vi "1D ARRAY TO 2D ARRAY.vi"() -> ()   [LabVIEW 2017]
panel:
  out "deleted portion":dbl[](array[numeric])
  out "array w/ subset deleted":dbl[](array[numeric])
  out "output array":dbl[](array[numeric])
  in  "new element/subarray":dbl
  out "subarray":dbl[](array[numeric])
  out "appended array":dbl[][](array[numeric])
  in  "Array 2":dbl[](array[numeric])
  in  "Array":dbl[](array[numeric])
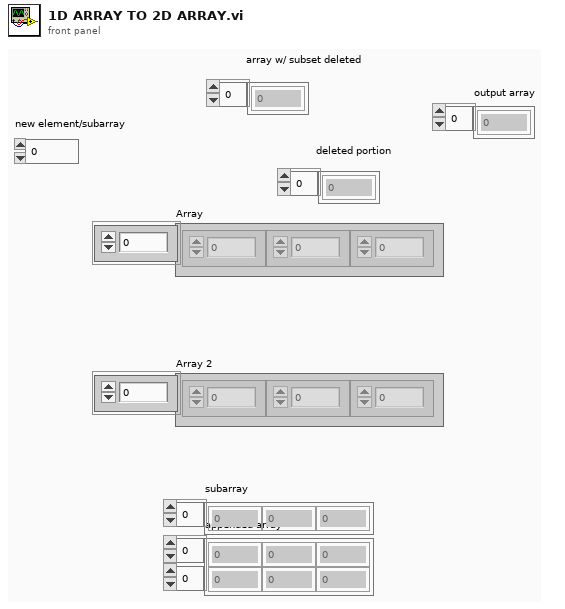
[diagram p1: front panel]
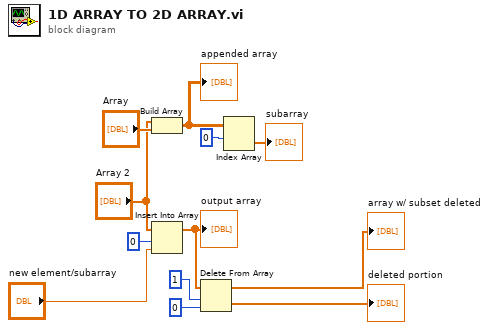
[diagram p0: block diagram]
diagram:
  n1 = Build Array("Array 2", "Array") -> (w10:dbl[][])
  "appended array" <- w10
  n2 = Insert Into Array(array="Array 2", index=0, new element="new element/subarray") -> (w5:dbl[])
  "output array" <- w5
  n3 = Delete From Array "Delete From Array"(array=w5, length=1, index=0) -> (deleted portion=→"deleted portion":dbl[], array with subset deleted=→"array w/ subset deleted":dbl[])
  n4 = Index Array(array=w10, index (row)=0 ("index")) -> (element=→"subarray":dbl[])  [unwired: 1 in]
